vi "Simple_Camram_Example.vi"() -> ()   [LabVIEW 2019]
uses:
  camera/Camera.lvclass
  <vilib>/picture/picture.llb/Draw 8-Bit Pixmap.vi
  <vilib>/picture/picture.llb/Draw True-Color Pixmap.vi
panel:
  out "colormap(U8)":u32[](array[numeric])
  out "Image(U16)":u16[][](graph)
  in  "Zoom [%]":i32(slide)=26 min=10 max=200 step=5 scale=10.0..200.0
  out "Image":picture
  out "rawImage":u16[][](array[numeric])
  in  "data_format":T1(ring)=enum."Mono16"
  in  "Image Index":u32 max=1145
  out "Recorded Images":u32
  in  "Quit":bool
  in  "roiY1":u64=2 min=2 max=1440 step=1
  in  "roiX1":u64=2 min=2 max=1920 step=1
  in  "roiY0":u64=1 min=1 max=1439 step=1
  in  "roiX0":u64=1 min=1 max=1919 step=1
  out "Image Height":u16
  out "Image Width":u16
  in  "segment":u16=1 caption="Segment" min=1 max=4
  out "Error":errorcluster {"code" format="%x"}
  # "This example shows for cameras with internal memory how to setup and record into a segment and show the images after record finished\nIt is a good starting point for writing own applications.\nBut it will not be fail save, i.e. doesnt react on errors, just handles them forward to the end\n\nUsage:\nSelect the segment you want to record into before you start the program.\nOnce started, the camera class will be initialized and images will be recorded automatically.\nWhen acquisition has finished you can address the images and set a certain roi \nTo finish the program click on quit application, this will force fan exit of the camera class"
  # "pco.labview"
  # "Camera Setup"
  # "Recording Control"
  # "Parameters for image readout"
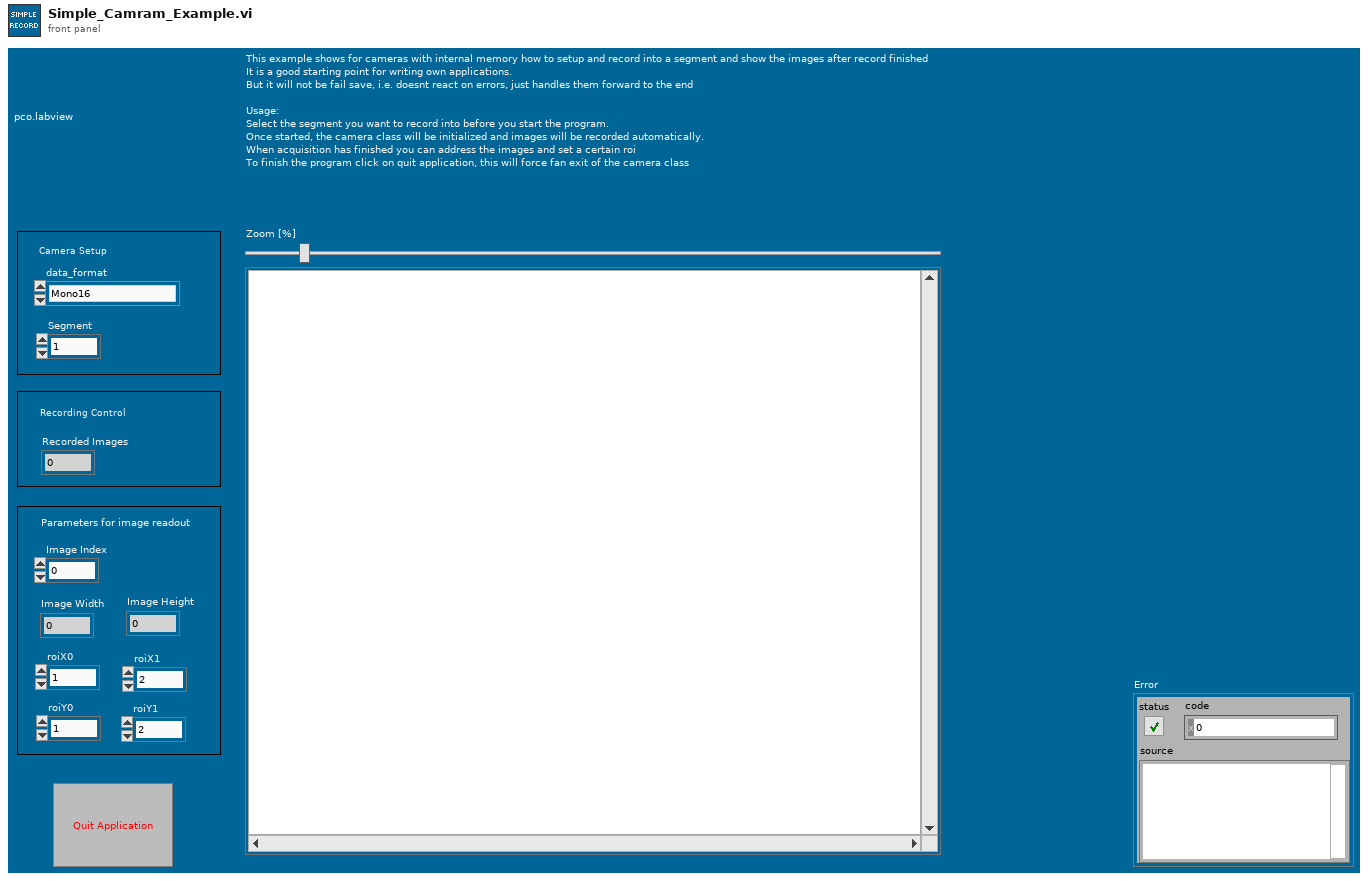
[diagram p1: front panel]
types:
  T1 = enum16{"Undefined", "Mono8", "Mono16", "BGRA8", "RGBA8", "BGRA16", "RGBA16", "CompressedMono8"}
  T2 = enum8{"Enabled", "Disabled", "Disabled and Grayed Out"}
  T3 = enum16{"sequence", "sequence non blocking", "ring buffer", "fifo", "tif", "multitif", "pcoraw", "b16", "dicom", "multidicom", "camram_ring", "camram_segment"}
  T4 = typedef "Camera.lvclass/binning.ctl" = cluster{"vert":u16, "horz":u16, "mode":u16}
  T5 = cluster{"exposure_time_s":dbl, "delay_time_s":dbl, "roi":cluster{"x0":u64, "y0":u64, "x1":u64, "y1":u64}, "timestamp_mode":u16, "pixelrate":u32, "conversion_factor":sgl, "trigger_mode":u16, "acquire_mode":u16, "acquire_sequence_number":u32, "metadata_mode":u16, "noisefilter_mode":u16, "pixel_format":u32, "binning":T4, "auto_exposure":cluster{"region":u16, "min_exposure_s":dbl, "max_exposure_s":dbl}}
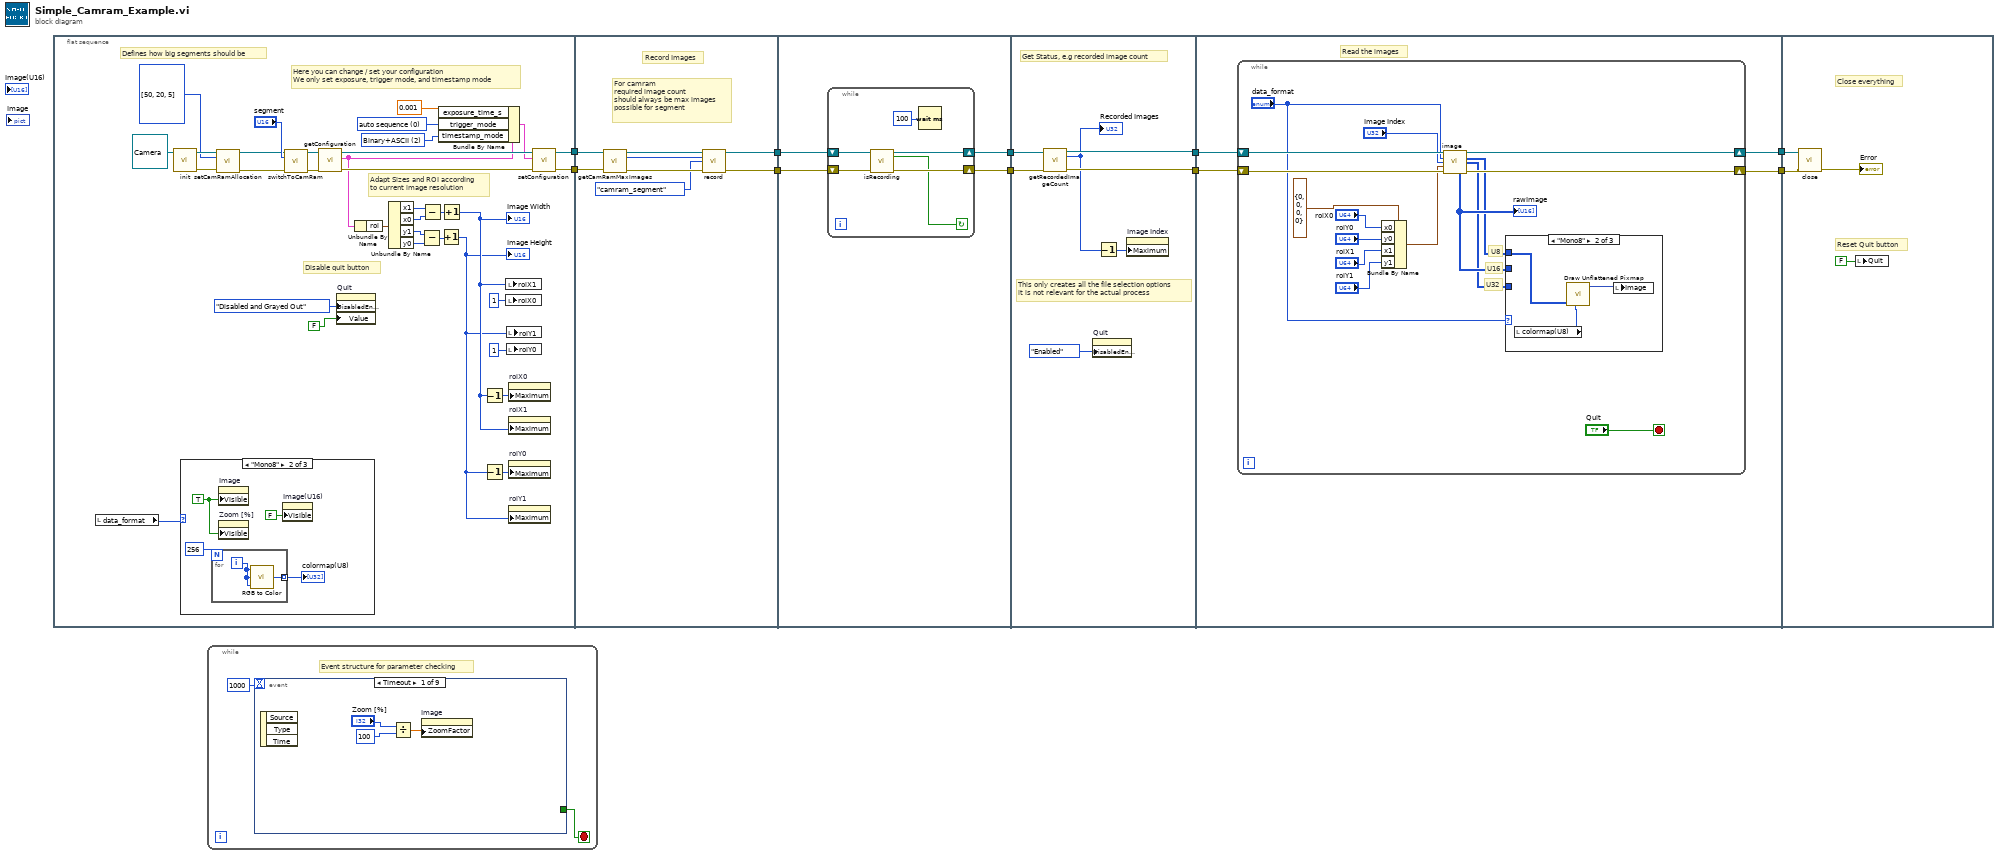
[diagram p0: block diagram]
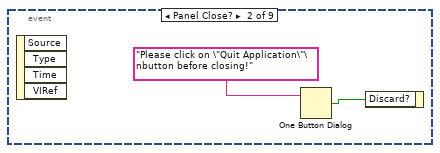
[diagram p2: hidden frame]
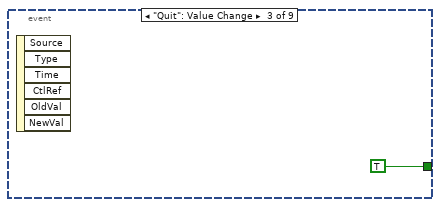
[diagram p3: hidden frame]
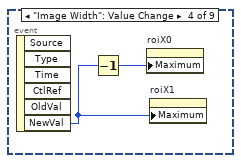
[diagram p4: hidden frame]
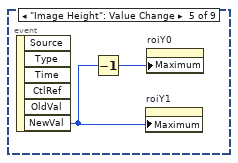
[diagram p5: hidden frame]
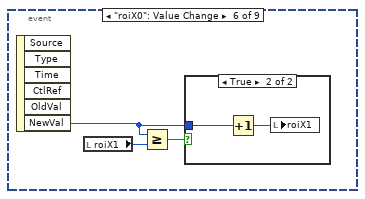
[diagram p6: hidden frame]
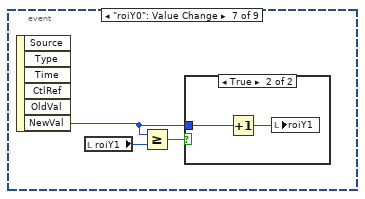
[diagram p8: hidden frame]
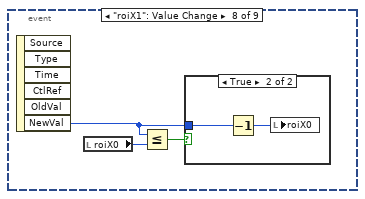
[diagram p10: hidden frame]
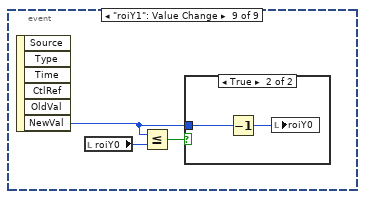
[diagram p12: hidden frame]
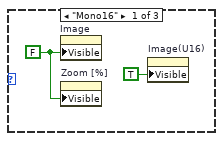
[diagram p14: hidden frame]
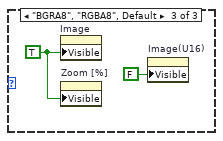
[diagram p15: hidden frame]
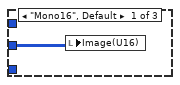
[diagram p16: hidden frame]
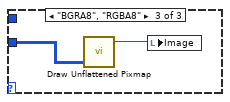
[diagram p17: hidden frame]
diagram:
  n1 = flat-sequence {
    tunnel: [w39] -> w10
    tunnel: [w38] -> w9
    tunnel: w10 -> [w60]
    tunnel: w9 -> [w59]
    tunnel: [w62] -> w4
    tunnel: [w61] -> w3
    tunnel: w4 -> [w66]
    tunnel: w3 -> [w65]
    tunnel: [w64] -> w2
    tunnel: [w63] -> w1
    tunnel: [w77] -> w8
    tunnel: [w76] -> w7
    tunnel: w2 -> [w79]
    tunnel: w1 -> [w78]
    tunnel: w8 -> [w82]
    tunnel: w7 -> [w83]
    tunnel: [w81] -> w6
    tunnel: [w80] -> w5
    tunnel: w6 -> [w107]
    tunnel: w5 -> [w106]
    frame #0 {
      w23 = u16 2 items=["OFF", "Binary", "Binary+ASCII", "ASCII"] ("TimestampMode")
      w43 = u16 0 items=["auto sequence"=0, "software trigger"=1, "external exposure start & software trigger"=2, "external exposure control"=3, "external synchronized"=4, "fast external exposure control"=5, "external CDS control"=6, "slow external exposure control"=7, "external synchronized HDSDI"=258] ("TriggerMode")
      # "Defines how big segments should be"
      # "Adapt Sizes and ROI according\nto current image resolution"
      # "Disable quit button"
      # "Here you can change / set your configuration\nWe only set exposure, trigger mode, and timestamp mode"
      n2 = local read "data_format"() -> (w20:T1)
      n3 = call-dynamic "init.vi"("Camera in"=refnum<class "Camera.lvclass"> refnum ("PCOCamera in")) -> ("Camera out"=w16:refnum<class "Camera.lvclass">, "error out"=w15:errorcluster)  [unwired: 8 in]
      n4 = case shown="\"Mono8\"" w20 {
        frame "Mono16" {
          w46 = FALSE ("Visible")
          n5 = property on="Image" class="Pict"("Visible"=w46) -> ()  [unwired: 2 in, 2 out]
          n6 = property on="Zoom [%]" class="Slide (strict)"("Visible"=w46) -> ()  [unwired: 2 in, 2 out]
          n7 = property on="Image(U16)" class="IntGraph (strict)"("Visible"=TRUE) -> ()  [unwired: 2 in, 2 out]
        }
        frame "Mono8" {
          w49 = TRUE ("Visible")
          n8 = for {
            N: 256 -> [_]
            tunnel: [w51] -> w48 mode=indexing
            i -> [w52]
            n9 = call <vilib>:"RGB to Color.vi"("B"=w52, "G"=w52, "R"=w52) -> ("Color"=w51:u32)
          }
          "colormap(U8)" <- w48
          n10 = property on="Image" class="Pict"("Visible"=w49) -> ()  [unwired: 2 in, 2 out]
          n11 = property on="Zoom [%]" class="Slide (strict)"("Visible"=w49) -> ()  [unwired: 2 in, 2 out]
          n12 = property on="Image(U16)" class="IntGraph (strict)"("Visible"=FALSE) -> ()  [unwired: 2 in, 2 out]
        }
        frame "BGRA8", "RGBA8", Default {
          w53 = TRUE ("Visible")
          n13 = property on="Image" class="Pict"("Visible"=w53) -> ()  [unwired: 2 in, 2 out]
          n14 = property on="Zoom [%]" class="Slide (strict)"("Visible"=w53) -> ()  [unwired: 2 in, 2 out]
          n15 = property on="Image(U16)" class="IntGraph (strict)"("Visible"=FALSE) -> ()  [unwired: 2 in, 2 out]
        }
      }
      n16 = call-dynamic "setCamRamAllocation.vi"("Camera in"=w16, "percents"=u32[] [50, 20, 5], "error in (no error)"=w15) -> ("Camera out"=w13:refnum<class "Camera.lvclass">, "error out"=w12:errorcluster)  [unwired: 11 in]
      n17 = call-dynamic "switchToCamRam.vi"("Camera in"=w13, "segment"="segment", "error in (no error)"=w12) -> ("Camera out"=w18:refnum<class "Camera.lvclass">, "error out"=w17:errorcluster)  [unwired: 11 in]
      n18 = call-dynamic "getConfiguration.vi"("error in (no error)"=w17, "Camera in"=w18) -> ("error out"=w41:errorcluster, "configuration"=w33:T5, "Camera out"=w42:refnum<class "Camera.lvclass">)  [unwired: 7 in]
      n19 = property on="Quit" class="Bool (strict)"("DisabledEnum"=T2."Disabled and Grayed Out" ("Disabled"), "Value"=FALSE ("Stop")) -> ()  [unwired: 2 in, 2 out]
      n20 = Unbundle By Name(w33) -> ("roi"=w32:cluster{"x0":u64, "y0":u64, "x1":u64, "y1":u64})
      n21 = Unbundle By Name(w32) -> ("x1"=w30:u64, "x0"=w31:u64, "y1"=w28:u64, "y0"=w29:u64)
      n22 = Subtract(x=w28, y=w29) -> (x-y=w26:u64)
      n23 = Subtract(x=w30, y=w31) -> (x-y=w27:u64)
      n24 = Bundle By Name(cluster=w33, "exposure_time_s"=0.001, "trigger_mode"=w43, "timestamp_mode"=w23) -> (w40:T5)
      n25 = Increment(x=w26) -> (x+1=w24:u64)
      "Image Height" <- w24
      n26 = Increment(x=w27) -> (x+1=w25:u64)
      "Image Width" <- w25
      n27 = Decrement(x=w25) -> (x-1=w35:u64)
      n28 = Decrement(x=w24) -> (x-1=w34:u64)
      n29 = local write "roiX1"(w25) -> ()
      n30 = local write "roiX0"(u16 1 ("roiY0")) -> ()
      n31 = local write "roiY1"(w24) -> ()
      n32 = local write "roiY0"(u16 1 ("roiY0")) -> ()
      n33 = property on="roiX0" class="DigNum (strict)"("Maximum"=w35) -> ()  [unwired: 2 in, 2 out]
      n34 = property on="roiX1" class="DigNum (strict)"("Maximum"=w25) -> ()  [unwired: 2 in, 2 out]
      n35 = property on="roiY0" class="DigNum (strict)"("Maximum"=w34) -> ()  [unwired: 2 in, 2 out]
      n36 = property on="roiY1" class="DigNum (strict)"("Maximum"=w24) -> ()  [unwired: 2 in, 2 out]
      n37 = call-dynamic "setConfiguration.vi"("error in (no error)"=w41, "configuration"=w40, "Camera in"=w42) -> ("error out"=w38:errorcluster, "Camera out"=w39:refnum<class "Camera.lvclass">)  [unwired: 7 in]
    }
    frame #1 {
      # "For camram\nrequired image count \nshould always be max images\npossible for segment"
      # "Record Images"
      n38 = call-dynamic "getCamRamMaxImages.vi"("Camera in"=w60, "error in (no error)"=w59) -> ("Camera out"=w58:refnum<class "Camera.lvclass">, "max_images"=w56:u32, "error out"=w57:errorcluster)  [unwired: 11 in]
      n39 = call-dynamic "record.vi"("Camera in"=w58, "num_images"=w56, "record_mode"=T3."camram_segment", "error in (no error)"=w57) -> ("Camera out"=w62:refnum<class "Camera.lvclass">, "error out"=w61:errorcluster)  [unwired: 10 in]
    }
    frame #2 {
      n40 = while {
        shift-right: [w70] -> w63
        shift-left: w65 -> [w71]
        shift-right: [w69] -> w64
        shift-left: w66 -> [w72]
        stop <- w67 continue-if-true
        n41 = call-dynamic "isRecording.vi"("Camera in"=w72, "error in (no error)"=w71) -> ("Camera out"=w69:refnum<class "Camera.lvclass">, "recording"=w67:bool, "error out"=w70:errorcluster)  [unwired: 11 in]
        n42 = Wait (ms)(milliseconds to wait=u32 100) -> ()  [unwired: 1 out]
      }
    }
    frame #3 {
      # "This only creates all the file selection options\nit is not relevant for the actual process"
      # "Get Status, e.g recorded image count"
      n43 = call-dynamic "getRecordedImageCount.vi"("Camera in"=w79, "error in (no error)"=w78) -> ("Camera out"=w77:refnum<class "Camera.lvclass">, "recorded_image_count"=w73:u32, "error out"=w76:errorcluster)  [unwired: 11 in]
      "Recorded Images" <- w73
      n44 = property on="Quit" class="Bool (strict)"("DisabledEnum"=T2."Enabled" ("Disabled")) -> ()  [unwired: 2 in, 2 out]
      n45 = Decrement(x=w73) -> (x-1=w74:u32)
      n46 = property on="Image Index" class="DigNum (strict)"("Maximum"=w74) -> ()  [unwired: 2 in, 2 out]
    }
    frame #4 {
      # "Read the images"
      n47 = while {
        shift-right: [w97] -> w81
        shift-left: w82 -> [w99]
        shift-right: [w92] -> w80
        shift-left: w83 -> [w98]
        stop <- "Quit" stop-if-true
        # "U32"
        # "U16"
        # "U8"
        n48 = Bundle By Name(cluster=cluster{"x0":u64, "y0":u64, "x1":u64, "y1":u64} {"x0"=0, "y0"=0, "x1"=0, "y1"=0} ("roi"), "x0"="roiX0", "y0"="roiY0", "x1"="roiX1", "y1"="roiY1") -> (w91:cluster{"x0":u64, "y0":u64, "x1":u64, "y1":u64})
        n49 = call-dynamic "image.vi"("Camera in"=w99, "data_format"="data_format", "image_index"="Image Index", "crop"=w91, "error in (no error)"=w98) -> ("Camera out"=w97:refnum<class "Camera.lvclass">, "image (U8)"=w84:u8[][], "image (U32)"=w85:u32[][], "raw_image (U16)"=w86:u16[][], "error out"=w92:errorcluster)  [unwired: 2 in, 4 out]
        "rawImage" <- w86
        n50 = case shown="\"Mono8\"" "data_format" {
          tunnel: w85 -> [_ _ w105]
          tunnel: w84 -> [_ w102 _]
          tunnel: w86 -> [w100 _ _]
          frame "Mono16", Default {
            n51 = local write "Image(U16)"(w100) -> ()
          }
          frame "Mono8" {
            n52 = local read "colormap(U8)"() -> (w101:u32[])
            n53 = call-poly <vilib>:"Draw Unflattened Pixmap.vi"("data"=w102, "color table"=w101) -> ("new picture"=w103:picture)  [unwired: 7 in]
            n54 = local write "Image"(w103) -> ()
          }
          frame "BGRA8", "RGBA8" {
            n55 = call-poly <vilib>:"Draw Unflattened Pixmap.vi"("data (RGB format)"=w105) -> ("new picture"=w104:picture)  [unwired: 8 in]
            n56 = local write "Image"(w104) -> ()
          }
        }
      }
    }
    frame #5 {
      # "Reset Quit button"
      # "Close everything"
      n57 = call-dynamic "close.vi"("error in (no error)"=w106, "Camera in"=w107) -> ("error out"=→"Error":errorcluster)  [unwired: 9 in]
      n58 = local write "Quit"(FALSE ("Stop")) -> ()
    }
  }
  n59 = while {
    stop <- w110 stop-if-true
    # "Event structure for parameter checking"
    n60 = event shown="[0] Timeout" {
      selector: _ -> [_ _ _ _ _ _ _ _ _]
      dyn-events: _ -> [_ _ _ _ _ _ _ _ _]
      timeout: 1000 -> [_ _ _ _ _ _ _ _ _]
      tunnel: [_ _ TRUE _ _ _ _ _ _] -> w110
      event Timeout {
        n61 = event-data() -> ()  [unwired: 1 in, 3 out]
        n62 = Divide(x="Zoom [%]", y=100 ("Zoom [%]")) -> (x/y=w112:dbl)
        n63 = property on="Image" class="Pict"("ZoomFactor"=w112) -> ()  [unwired: 2 in, 2 out]
      }
      event Panel Close? {
        n64 = event-data() -> ()  [unwired: 1 in, 4 out]
        n65 = One Button Dialog(message="Please click on \"Quit Application\"\nbutton before closing!") -> (true=w115:bool)  [unwired: 1 in]
        n66 = event-data("Discard?"=w115) -> ()  [unwired: 1 in, 1 out]
      }
      event "Quit": Value Change {
        n67 = event-data() -> ()  [unwired: 1 in, 6 out]
      }
      event "Image Width": Value Change {
        n68 = event-data() -> ("NewVal"=w118:u16)  [unwired: 1 in, 5 out]
        n69 = Decrement(x=w118) -> (x-1=w119:u16)
        n70 = property on="roiX0" class="DigNum (strict)"("Maximum"=w119) -> ()  [unwired: 2 in, 2 out]
        n71 = property on="roiX1" class="DigNum (strict)"("Maximum"=w118) -> ()  [unwired: 2 in, 2 out]
      }
      event "Image Height": Value Change {
        n72 = event-data() -> ("NewVal"=w120:u16)  [unwired: 1 in, 5 out]
        n73 = Decrement(x=w120) -> (x-1=w121:u16)
        n74 = property on="roiY1" class="DigNum (strict)"("Maximum"=w120) -> ()  [unwired: 2 in, 2 out]
        n75 = property on="roiY0" class="DigNum (strict)"("Maximum"=w121) -> ()  [unwired: 2 in, 2 out]
      }
      event "roiX0": Value Change {
        n76 = event-data() -> ("NewVal"=w122:u64)  [unwired: 1 in, 5 out]
        n77 = local read "roiX1"() -> (w124:u64)
        n78 = Greater Or Equal?(x=w122, y=w124) -> (x >= y?=w123:bool)
        n79 = case shown="True" w123 {
          tunnel: w122 -> [_ w126]
          frame False {
          }
          frame True {
            n80 = Increment(x=w126) -> (x+1=w125:u64)
            n81 = local write "roiX1"(w125) -> ()
          }
        }
      }
      event "roiY0": Value Change {
        n82 = event-data() -> ("NewVal"=w127:u64)  [unwired: 1 in, 5 out]
        n83 = local read "roiY1"() -> (w129:u64)
        n84 = Greater Or Equal?(x=w127, y=w129) -> (x >= y?=w128:bool)
        n85 = case shown="True" w128 {
          tunnel: w127 -> [_ w131]
          frame False {
          }
          frame True {
            n86 = Increment(x=w131) -> (x+1=w130:u64)
            n87 = local write "roiY1"(w130) -> ()
          }
        }
      }
      event "roiX1": Value Change {
        n88 = event-data() -> ("NewVal"=w132:u64)  [unwired: 1 in, 5 out]
        n89 = local read "roiX0"() -> (w134:u64)
        n90 = Less Or Equal?(x=w132, y=w134) -> (x <= y?=w133:bool)
        n91 = case shown="True" w133 {
          tunnel: w132 -> [_ w136]
          frame False {
          }
          frame True {
            n92 = Decrement(x=w136) -> (x-1=w135:u64)
            n93 = local write "roiX0"(w135) -> ()
          }
        }
      }
      event "roiY1": Value Change {
        n94 = event-data() -> ("NewVal"=w137:u64)  [unwired: 1 in, 5 out]
        n95 = local read "roiY0"() -> (w139:u64)
        n96 = Less Or Equal?(x=w137, y=w139) -> (x <= y?=w138:bool)
        n97 = case shown="True" w138 {
          tunnel: w137 -> [_ w141]
          frame False {
          }
          frame True {
            n98 = Decrement(x=w141) -> (x-1=w140:u64)
            n99 = local write "roiY0"(w140) -> ()
          }
        }
      }
    }
  }
